vi "AnalizaDatos.vi"() -> ()   [LabVIEW 2013]
uses:
  <vilib>/Utility/file.llb/Read From Spreadsheet File (DBL).vi
  <vilib>/measure/maspectr.llb/FFT Spectrum (Mag-Phase) for 1 Chan.vi
  <vilib>/measure/NI_MAPro.lvlib
panel:
  out "spectrum units table 2":string[][](table)=[["FFT", "N * V", "N/2 * Vpk"], ["Power Spectrum", "V^2", "1/2 * Vrms^2"], ["Auto Power Spectrum", "V^2", "Vrms^2"], ["Amplitude and Phase Spectrum", "V", "Vrms"], ["FFT Power Spectrum", "V^2", "Vrms^2"], ["FFT Power Spectral Density", "V^2/Hz", "Vrms^2/Hz"], ["FFT Spectrum (Mag-Phase)", "V", "Vrms"], ["FFT Spectrum (Real-Imag)", "V", "Vrms"]]
  out "max index(es) 2":i32
  out "Max freq 2":dbl
  out "max frec value 2":dbl
  out "FFT 2":waveform(dbl)(graph)
  out "df 2":dbl
  out "f0 2":dbl
  out "spectrum units table":string[][](table)=[["FFT", "N * V", "N/2 * Vpk"], ["Power Spectrum", "V^2", "1/2 * Vrms^2"], ["Auto Power Spectrum", "V^2", "Vrms^2"], ["Amplitude and Phase Spectrum", "V", "Vrms"], ["FFT Power Spectrum", "V^2", "Vrms^2"], ["FFT Power Spectral Density", "V^2/Hz", "Vrms^2/Hz"], ["FFT Spectrum (Mag-Phase)", "V", "Vrms"], ["FFT Spectrum (Real-Imag)", "V", "Vrms"]]
  out "max index(es)":i32
  out "Max freq":dbl
  out "max frec value":dbl
  out "FFT":waveform(dbl)(graph)
  out "df":dbl
  out "f0":dbl
  out "Multiple Updates (Multiple Plots)":cluster{dbl, dbl}[](graph)
  out "Entrada Centrada en cero":waveform(dbl)(graph)
  out "Entrada con Offset":waveform(dbl)(graph)
  out "Salida Centrada en cero":waveform(dbl)(graph)
  in  "Elementos a eliminar":i32
  in  "Periodo de muestreo (segundos)":dbl=0.05
  out "Salida con Offset":waveform(dbl)(graph)
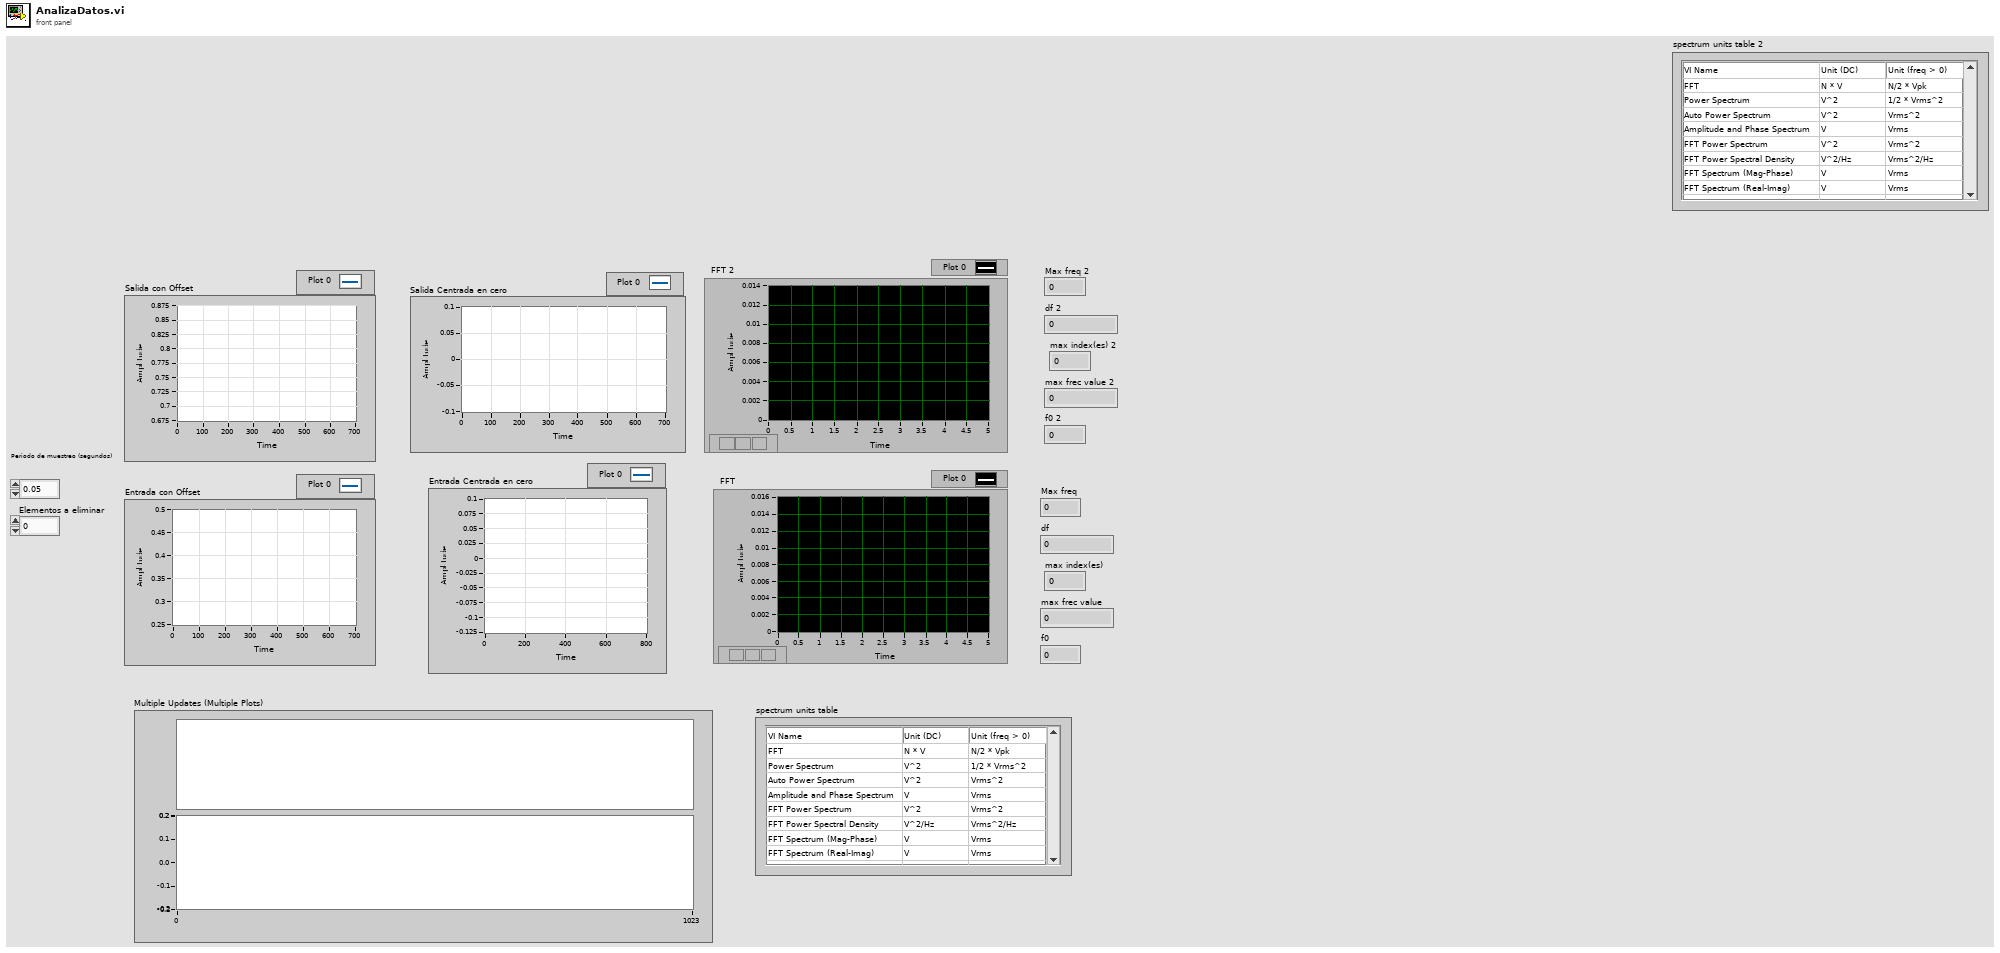
[diagram p1: front panel]
types:
  T1 = cluster{"dB On (F)":bool, "unwrap phase (F)":bool, "convert to degree (F)":bool}
  T2 = enum16{"None ", "Hanning", "Hamming", "Blackman-Harris", "Exact Blackman", "Blackman", "Flat Top", "4 Term B-Harris ", "7 Term B-Harris", "Low Sidelobe"}
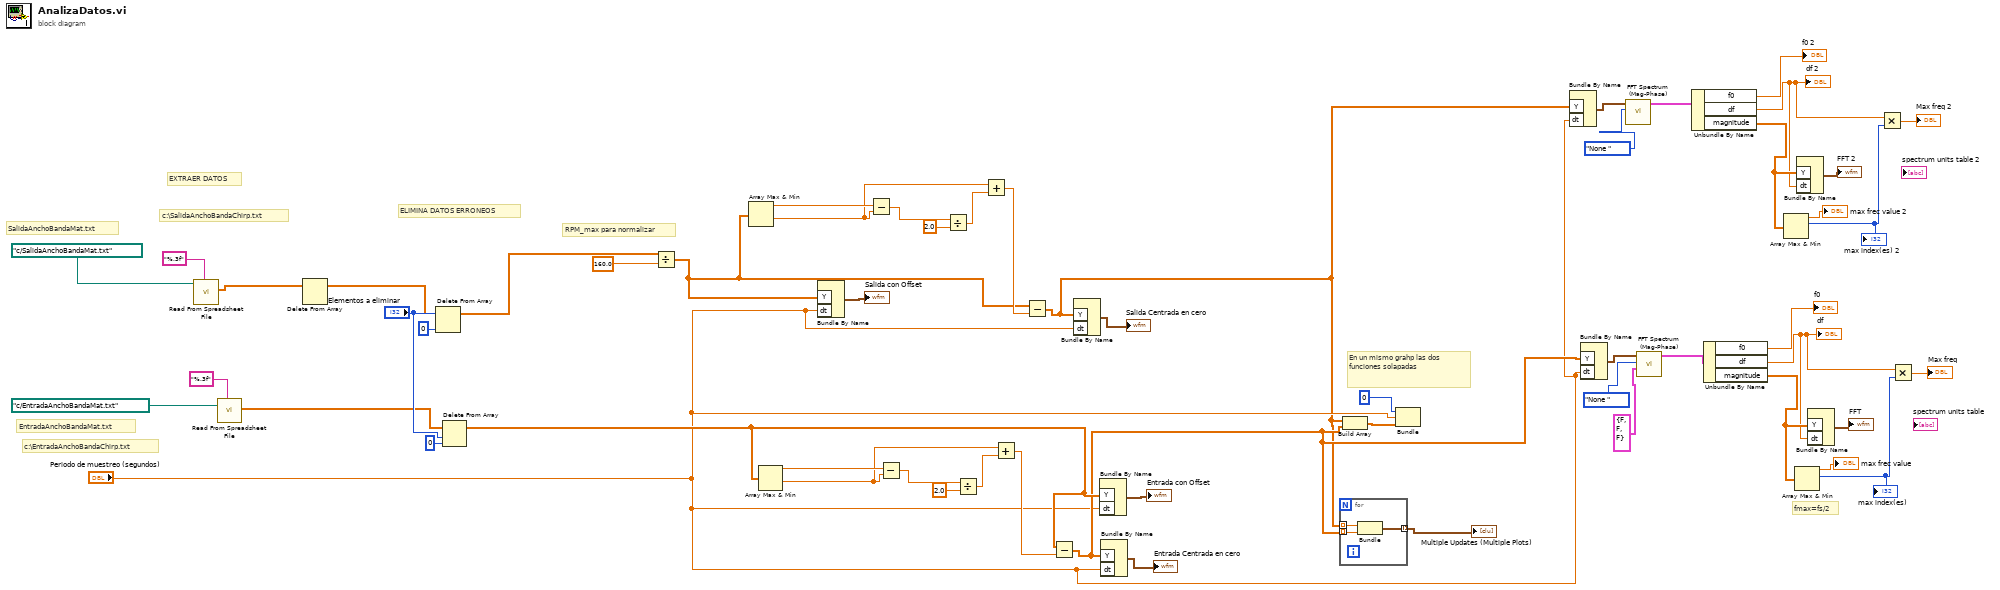
[diagram p0: block diagram]
diagram:
  # "c:\\SalidaAnchoBandaChirp.txt"
  # "c:\\EntradaAnchoBandaChirp.txt"
  # "fmax=fs/2"
  # "SalidaAnchoBandaMat.txt"
  # "EntradaAnchoBandaMat.txt"
  # "En un mismo grahp las dos funciones solapadas"
  # "ELIMINA DATOS ERRONEOS"
  # "EXTRAER DATOS"
  # "RPM_max para normalizar"
  n1 = call-poly <vilib>:"Read From Spreadsheet File.vi"("format (%.3f)"="%.3f", "file path (dialog if empty)"=path "c:/SalidaAnchoBandaMat.txt") -> ("first row"=w2:dbl[])  [unwired: 5 in, 4 out]
  n2 = call-poly <vilib>:"Read From Spreadsheet File.vi"("format (%.3f)"="%.3f" ("format string"), "file path (dialog if empty)"=path "c:/EntradaAnchoBandaMat.txt") -> ("first row"=w4:dbl[])  [unwired: 5 in, 4 out]
  n3 = Delete From Array(array=w2) -> (array with subset deleted=w1:dbl[])  [unwired: 2 in, 1 out]
  n4 = Delete From Array(array=w1, length="Elementos a eliminar", index=0) -> (array with subset deleted=w52:dbl[])  [unwired: 1 out]
  n5 = Delete From Array(array=w4, length="Elementos a eliminar", index=0) -> (array with subset deleted=w37:dbl[])  [unwired: 1 out]
  n6 = Divide(x=w52, y=160.0 ("max rpm")) -> (x/y=w35:dbl[])
  n7 = Array Max & Min(array=w35) -> (max value=w49:dbl, min value=w48:dbl)  [unwired: 2 out]
  n8 = Array Max & Min(array=w37) -> (max value=w42:dbl, min value=w41:dbl)  [unwired: 2 out]
  n9 = Bundle By Name("Y"=w35, "dt"="Periodo de muestreo (segundos)") -> (→"Salida con Offset":waveform(dbl))  [unwired: 1 in]
  n10 = Subtract(x=w49, y=w48) -> (x-y=w47:dbl)
  n11 = Subtract(x=w42, y=w41) -> (x-y=w40:dbl)
  n12 = Divide(x=w47, y=2.0) -> (x/y=w45:dbl)
  n13 = Divide(x=w40, y=2.0) -> (x/y=w38:dbl)
  n14 = Add(x=w48, y=w45) -> (x+y=w44:dbl)
  n15 = Add(x=w41, y=w38) -> (x+y=w36:dbl)
  n16 = Subtract(x=w35, y=w44) -> (x-y=w11:dbl[])
  n17 = Subtract(x=w37, y=w36) -> (x-y=w23:dbl[])
  n18 = Bundle By Name("Y"=w11, "dt"="Periodo de muestreo (segundos)") -> (→"Salida Centrada en cero":waveform(dbl))  [unwired: 1 in]
  n19 = Bundle By Name("Y"=w37, "dt"="Periodo de muestreo (segundos)") -> (→"Entrada con Offset":waveform(dbl))  [unwired: 1 in]
  n20 = Bundle By Name("Y"=w23, "dt"="Periodo de muestreo (segundos)") -> (→"Entrada Centrada en cero":waveform(dbl))  [unwired: 1 in]
  n21 = for {
    tunnel: w11 -> [w60] mode=indexing
    tunnel: w23 -> [w59] mode=indexing
    tunnel: [w58] -> w32 mode=indexing
    n22 = Bundle(w60, w59) -> (w58:cluster{dbl, dbl})  [unwired: 1 in]
  }
  "Multiple Updates (Multiple Plots)" <- w32
  n23 = Build Array(w11, w23) -> (w56:dbl[][])
  n24 = Bundle(0, "Periodo de muestreo (segundos)"="Periodo de muestreo (segundos)", w56) -> ()  [unwired: 1 in, 1 out]
  n25 = Bundle By Name("Y"=w11, "dt"="Periodo de muestreo (segundos)") -> (w13:waveform(dbl))  [unwired: 1 in]
  n26 = Bundle By Name("Y"=w23, "dt"="Periodo de muestreo (segundos)") -> (w22:waveform(dbl))  [unwired: 1 in]
  n27 = call-poly <vilib>:"FFT Spectrum (Mag-Phase).vi"("window"=T2."None ", "time signal"=w13) -> ("magnitude"=w21:cluster{"f0":dbl, "df":dbl, "magnitude":dbl[]})  [unwired: 5 in, 4 out]
  n28 = call-poly <vilib>:"FFT Spectrum (Mag-Phase).vi"("view"=T1 {"dB On (F)"=FALSE, "unwrap phase (F)"=FALSE, "convert to degree (F)"=FALSE}, "window"=T2."None ", "time signal"=w22) -> ("magnitude"=w31:cluster{"f0":dbl, "df":dbl, "magnitude":dbl[]})  [unwired: 4 in, 4 out]
  n29 = Unbundle By Name(w21) -> ("f0"=→"f0 2":dbl, "df"=w14:dbl, "magnitude"=w18:dbl[])
  "df 2" <- w14
  n30 = Unbundle By Name(w31) -> ("f0"=→"f0":dbl, "df"=w24:dbl, "magnitude"=w28:dbl[])
  "df" <- w24
  n31 = Array Max & Min(array=w18) -> (max value=→"max frec value 2":dbl, max index (indices)=w16:i32)  [unwired: 2 out]
  "max index(es) 2" <- w16
  n32 = Array Max & Min(array=w28) -> (max value=→"max frec value":dbl, max index (indices)=w26:i32)  [unwired: 2 out]
  "max index(es)" <- w26
  n33 = Bundle By Name("Y"=w18, "dt"=w14) -> (→"FFT 2":waveform(dbl))  [unwired: 1 in]
  n34 = Bundle By Name("Y"=w28, "dt"=w24) -> (→"FFT":waveform(dbl))  [unwired: 1 in]
  n35 = Multiply(x=w14, y=w16) -> (x*y=→"Max freq 2":dbl)
  n36 = Multiply(x=w24, y=w26) -> (x*y=→"Max freq":dbl)
